vi "Xsens Main Process (VISA) (TESTER).vi"() -> (0 "error out":errorcluster)   [LabVIEW 2019]
doc: "This is the RT top level decoder, parser, and data save API for the XSens MTI 710 INS. It contains several subvis that perform the following functions:\n1. Copy measurement data from the VISA serial port read message queue\n2. Perform a checksum on the received data\n3. Inspect the data packet, extracting the data types, byte counts, and data payload into an array\n4. Parse the data types and decode the HEX\n5. Save each message to TDMS file(s)\n\n2020 NREL"
uses:
  Globals and Definitions/Serial - Settings.ctl
  Globals and Definitions/Initialization Globals.vi
  Globals and Definitions/RT Globals RD v1.0.vi
panel:
  out "Q In":string
  out "VISA Read Error":errorcluster
  out "INS":string[][](array[string])
  out "GNSS":string[][](array[string])
  out "CS Good":bool
  out "All Msg Sizes (Local)":string[](array[string])
  out "Sorted DTs (Local)":string[](array[string])
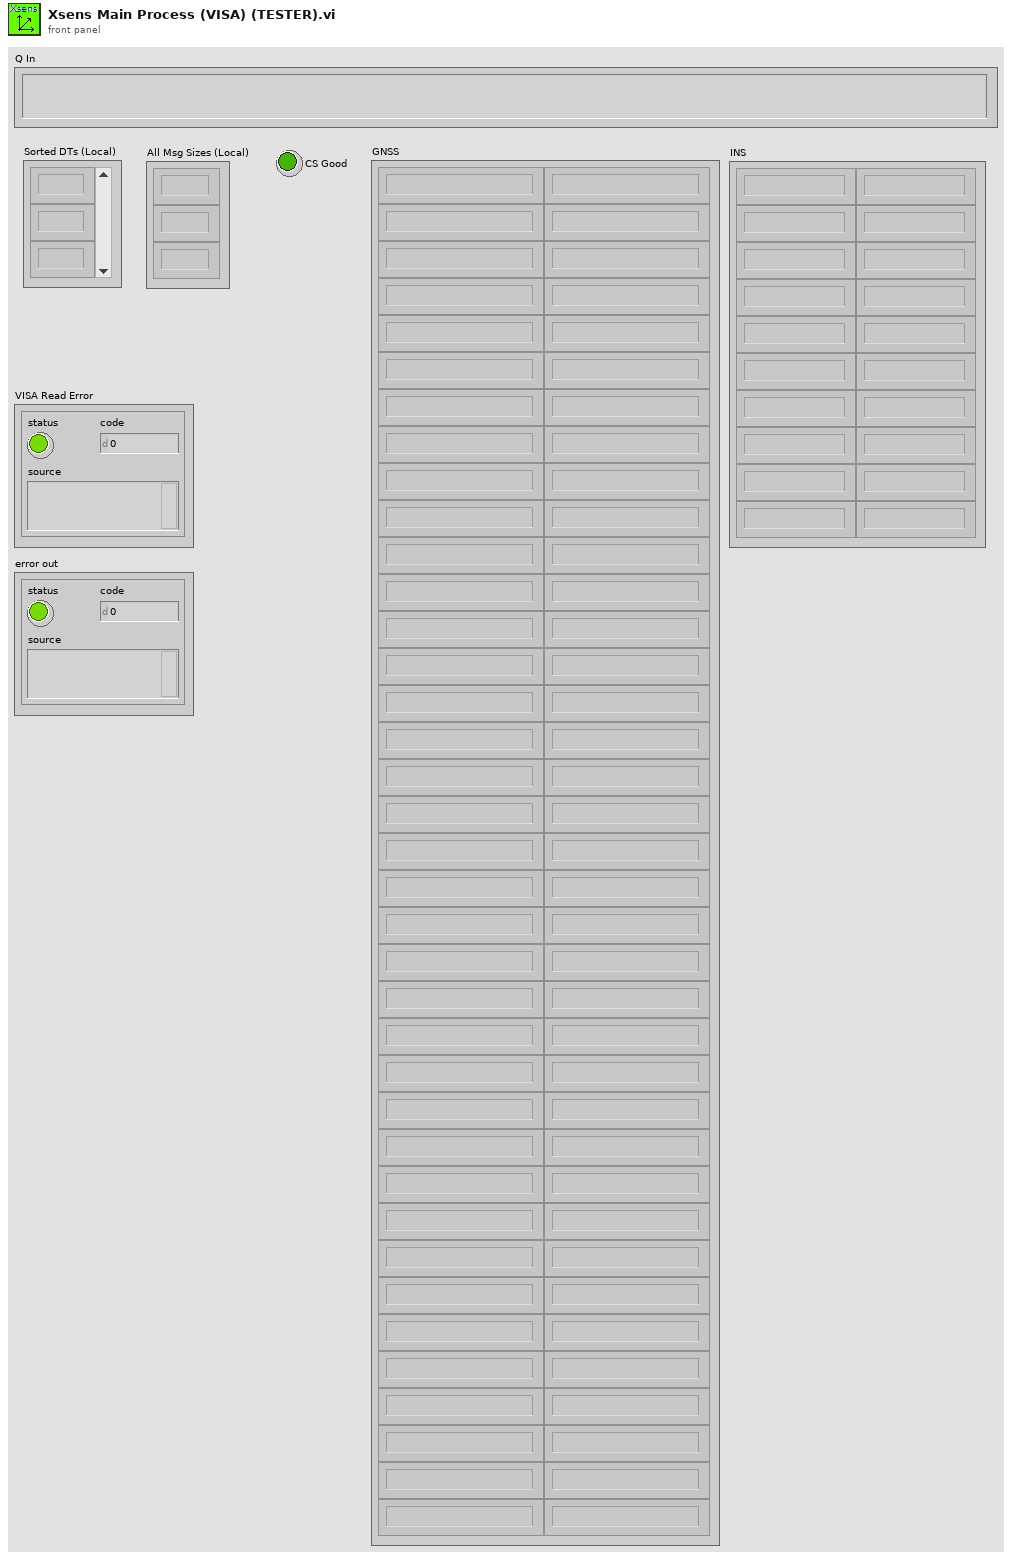
[diagram p1: front panel]
types:
  T1 = typedef "Serial - Settings.ctl" = cluster{"baud rate":u32, "data bits":u16, "parity":enum16{"None", "Odd", "Even", "Mark", "Space"}, "stop bits":u16, "flow control":u16}
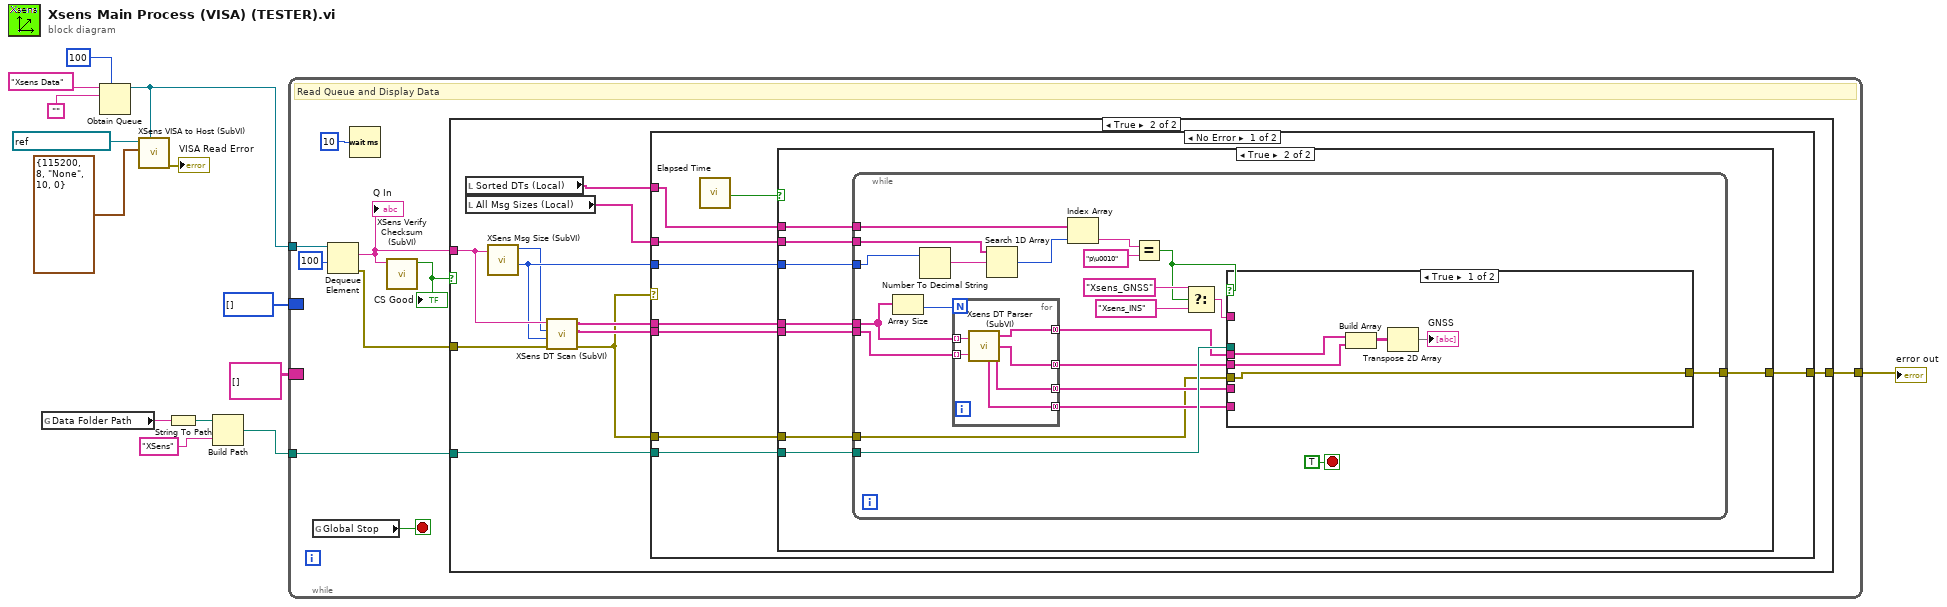
[diagram p0: block diagram]
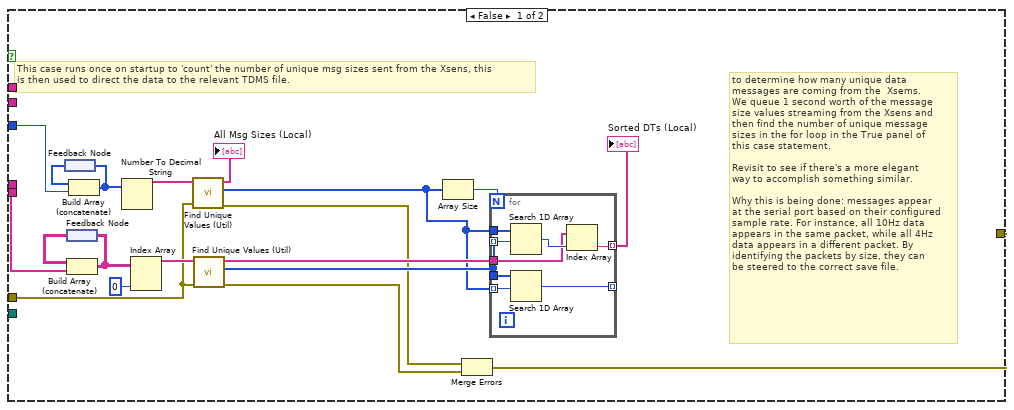
[diagram p3: hidden frame]
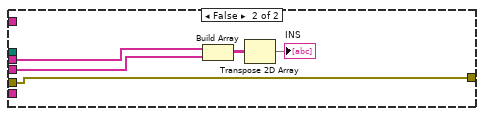
[diagram p4: hidden frame]
diagram:
  n1 = global read "Initialization Globals.vi" "Data Folder Path"() -> (w10:string)
  n2 = Obtain Queue(max queue size (-1, unlimited)=100, name (unnamed)="Xsens Data", element data type="") -> (queue out=w5:refnum<queue>)  [unwired: 2 in, 2 out]
  n3 = call "XSens VISA to Host (SubVI).vi"("XSense Queue In"=w5, "Serial Settings"=T1 {"baud rate"=115200, "data bits"=8, "parity"=enum."None", "stop bits"=10, "flow control"=0}, "VISA resource name"=refnum<visa-resource-name> "ASRL3::INSTR") -> ("error out"=→"VISA Read Error":errorcluster)  [unwired: 8 in]
  n4 = String To Path(string=w10) -> (path=w11:path)
  n5 = Build Path(base path=w11, name or relative path="XSens") -> (appended path=w9:path)
  n6 = while {
    tunnel: w9 -> [w21]
    border: string[][] [] -> [_]
    border: u16[] [] -> [_]
    tunnel: w5 -> [w20]
    tunnel: [w17] -> w7
    stop <- w16 stop-if-true
    # "Read Queue and Display Data"
    n7 = global read "RT Globals RD v1.0.vi" "Global Stop"() -> (w16:bool)
    n8 = Dequeue Element(queue=w20, timeout in ms (-1)=100) -> (element=w15:string, error out=w18:errorcluster)  [unwired: 1 in, 2 out]
    "Q In" <- w15
    n9 = Wait (ms)(milliseconds to wait=u32 10) -> ()  [unwired: 1 out]
    n10 = call "XSens Verify Checksum (SubVI).vi"("MTData2 Msg"=w15) -> ("CS Good?"=w22:bool)  [unwired: 10 in]
    "CS Good" <- w22
    n11 = case shown="True" w22 {
      tunnel: w15 -> [_ w33]
      tunnel: w21 -> [_ w35]
      tunnel: w18 -> [w24 w30]
      tunnel: [w24 w34] -> w17
      frame False {
      }
      frame True {
        n12 = local read "Sorted DTs (Local)"() -> (w26:string[])
        n13 = local read "All Msg Sizes (Local)"() -> (w25:string[])
        n14 = call "XSens Msg Size (SubVI).vi"("From Q"=w33) -> ("Data Size"=w28:u16, "Index"=w27:i16)  [unwired: 9 in]
        n15 = call "XSens DT Scan (SubVI).vi"("string in"=w33, "Index"=w27, "Payload Size"=w28, "Error In"=w30) -> ("DT Out"=w32:string[], "DT String"=w31:string[], "Error Out"=w29:errorcluster)  [unwired: 2 in]
        n16 = case shown="No Error" w29 {
          selector: w29 -> [_ w118]
          tunnel: w35 -> [w43 _]
          tunnel: w29 -> [w42 _]
          tunnel: [w41 w118] -> w34
          tunnel: w32 -> [w40 _]
          tunnel: w31 -> [w39 _]
          tunnel: w28 -> [w38 _]
          tunnel: w26 -> [w37 _]
          tunnel: w25 -> [w36 _]
          frame No Error {
            n17 = call "Elapsed Time"() -> ("Time has Elapsed"=w44:bool)  [unwired: 12 in, 7 out]
            n18 = case shown="True" w44 {
              tunnel: w40 -> [w53 w79]
              tunnel: w39 -> [_ w78]
              tunnel: w38 -> [w61 w77]
              tunnel: w43 -> [_ w76]
              tunnel: w42 -> [w47 w75]
              tunnel: [w48 w74] -> w41
              tunnel: w37 -> [_ w73]
              tunnel: w36 -> [_ w72]
              frame False {
                # "This case runs once on startup to 'count' the number of unique msg sizes sent from the Xsens, this\nis then used to direct the data to the relevant TDMS file."
                # "to determine how many unique data\nmessages are coming from the  Xsems.\nWe queue 1 second worth of the message\nsize values streaming from the Xsens and\nthen find the number of unique message\nsizes in the for loop in the True panel of \nthis case statement. \n\nRevisit to see if there's a more elegant \nway to accomplish something similar.\n\nWhy this is being done: messages appear\nat the serial port based on their configured\nsample rate. For instance, all 10Hz data\nappears in the same packet, while all 4Hz\ndata appears in a different packet. By \nidentifying the packets by size, they can \nbe steered to the correct save file."
                n19 = feedback #1() -> (w60:u16[])
                n20 = feedback #2() -> (w63:string[][])
                n21 = Build Array (concatenate)(w63, w53) -> (w52:string[][])
                n22 = feedback-in #2(w52) -> ()
                n23 = Build Array (concatenate)(w60, w61) -> (w59:u16[])
                n24 = feedback-in #1(w59) -> ()
                n25 = Number To Decimal String(number=w59) -> (decimal integer string=w51:string[])  [unwired: 1 in]
                n26 = Index Array(array=w52, index (col)=0 ("disabled index (col)")) -> (element=w54:string[])  [unwired: 1 in]
                n27 = call "Find Unique Values (Util).vi"("error in (no error)"=w47, "Array in"=w51) -> ("error out"=w46:errorcluster, "Number repeats for each"=w49:i32[], "Unique Values"=→"All Msg Sizes (Local)":string[])  [unwired: 7 in]
                n28 = call "Find Unique Values (Util).vi"("error in (no error)"=w47, "Array in"=w54) -> ("error out"=w45:errorcluster, "Number repeats for each"=w57:i32[], "Unique Values"=w56:string[])  [unwired: 7 in]
                n29 = Array Size(array=w49) -> (size(s)=w58:i32)
                n30 = Merge Errors(w46, w45) -> (w48:errorcluster)
                n31 = for {
                  N: w58 -> [_]
                  tunnel: w49 -> [w71]
                  tunnel: w57 -> [w70]
                  tunnel: w49 -> [w69] mode=indexing
                  tunnel: w57 -> [w68] mode=indexing
                  tunnel: [w67] -> _ mode=indexing
                  tunnel: w56 -> [w65]
                  tunnel: [w64] -> w55 mode=indexing
                  n32 = Search 1D Array(1D array=w71, element=w68) -> (index of element=w66:i32)  [unwired: 1 in]
                  n33 = Search 1D Array(1D array=w70, element=w69) -> (index of element=w67:i32)  [unwired: 1 in]
                  n34 = Index Array(array=w65, index=w66) -> (element=w64:string)
                }
                "Sorted DTs (Local)" <- w55
              }
              frame True {
                n35 = while {
                  tunnel: w79 -> [w101]
                  tunnel: w78 -> [w100]
                  tunnel: w77 -> [w92]
                  tunnel: w76 -> [w97]
                  tunnel: w75 -> [w83]
                  tunnel: [w82] -> w74
                  tunnel: w73 -> [w81]
                  tunnel: w72 -> [w80]
                  stop <- TRUE stop-if-true
                  n36 = Array Size(array=w101) -> (size(s)=w98:i32)
                  n37 = Number To Decimal String(number=w92) -> (decimal integer string=w91:string)  [unwired: 1 in]
                  n38 = for {
                    N: w98 -> [_]
                    tunnel: w101 -> [w117] mode=indexing
                    tunnel: w100 -> [w116] mode=indexing
                    tunnel: [w114] -> w95 mode=concatenating
                    tunnel: [w115] -> w96 mode=concatenating
                    tunnel: [w113] -> w94 mode=concatenating
                    tunnel: [w112] -> w93 mode=concatenating
                    n39 = call "Xsens DT Parser (SubVI).vi"("DT String In"=w116, "DataType In"=w117) -> ("Channel Units"=w113:string[], "Channel DataTypes"=w112:string[], "Decoded Data Out"=w114:string[], "Channel Names"=w115:string[])  [unwired: 1 in]
                  }
                  n40 = Search 1D Array(1D array=w80, element=w91) -> (index of element=w90:i32)  [unwired: 1 in]
                  n41 = Index Array(array=w81, index=w90) -> (element=w88:string)
                  n42 = Equal?(x=w88, y="p\u0010") -> (x = y?=w84:bool)
                  n43 = Select(t="Xsens_GNSS" ("group name"), s=w84, f="Xsens_INS" ("group name")) -> (s? t:f=w85:string)
                  n44 = case shown="True" w84 {
                    tunnel: w97 -> [_ _]
                    tunnel: w96 -> [w105 w111]
                    tunnel: w95 -> [w104 w110]
                    tunnel: w94 -> [_ _]
                    tunnel: w93 -> [_ _]
                    tunnel: w85 -> [_ _]
                    tunnel: w83 -> [w103 w108]
                    tunnel: [w103 w108] -> w82
                    frame True {
                      n45 = Build Array(w105, w104) -> (w106:string[][])
                      n46 = Transpose 2D Array(2D array=w106) -> (transposed array=→"GNSS":string[][])
                    }
                    frame False {
                      n47 = Build Array(w111, w110) -> (w109:string[][])
                      n48 = Transpose 2D Array(2D array=w109) -> (transposed array=→"INS":string[][])
                    }
                  }
                }
              }
            }
          }
          frame Error {
          }
        }
      }
    }
  }
  "error out" <- w7
